vi "Formula_6.1.vi"(6 "x":i32=2, 7 "t_aus":i32, 8 "t":i32, 10 "K_last":dbl, 11 "K_vor":dbl) -> (2 "K_Gr":dbl)   [LabVIEW 2015]
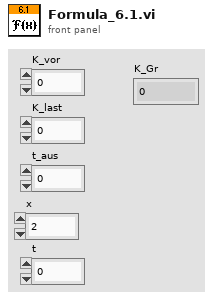
[diagram p1: front panel]
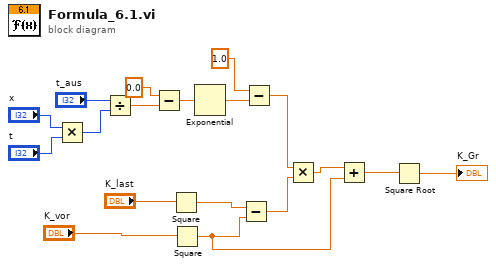
[diagram p0: block diagram]
diagram:
  n1 = Multiply(x="x", y="t") -> (x*y=w13:i32)
  n2 = Divide(x="t_aus", y=w13) -> (x/y=w12:dbl)
  n3 = Subtract(x=0.0, y=w12) -> (x-y=w10:dbl)
  n4 = Square(x="K_last") -> (x^2=w17:dbl)
  n5 = Square(x="K_vor") -> (x^2=w2:dbl)
  n6 = Exponential(1:w10) -> (0:w8:dbl)
  n7 = Subtract(x=w17, y=w2) -> (x-y=w16:dbl)
  n8 = Subtract(x=1.0, y=w8) -> (x-y=w4:dbl)
  n9 = Multiply(x=w4, y=w16) -> (x*y=w3:dbl)
  n10 = Add(x=w3, y=w2) -> (x+y=w1:dbl)
  n11 = Square Root(x=w1) -> (sqrt(x)=→"K_Gr":dbl)
